vi "MultithreadedUDPReadWriteAnalyze.vi"() -> ()   [LabVIEW 2012]
panel:
  out "regmap":string
  out "power monitoring \ndata string":string
  out "UDP Send Error Initialize":errorcluster
  out "Fresh Register map":bool
  out "Last Command Sent":string
  out "UDP Send Error":errorcluster
  out "Original Register Map":string
  out "Register Map":string
  in  "stop":bool
  out "NumBins":u32
  out "Cnts/Bin":u32
  out "Prof/Hist":u32
  out "Sync":u32
  out "Channel":u32
  out "rTime":u32
  out "frameCntr":u32
  out "UDP Close Error":errorcluster
  out "Profile Byte by Byte":u8[](graph)
  out "Profile":u32[](graph)
  in  "Profile Number":u32=1
  out "Queue close error":errorcluster
  out "Queue Add Data Error":errorcluster
  out "Queue creation error":errorcluster
  out "UDP Read Error":errorcluster
  in  "port":u16=300
  out "UDP Open Error":errorcluster
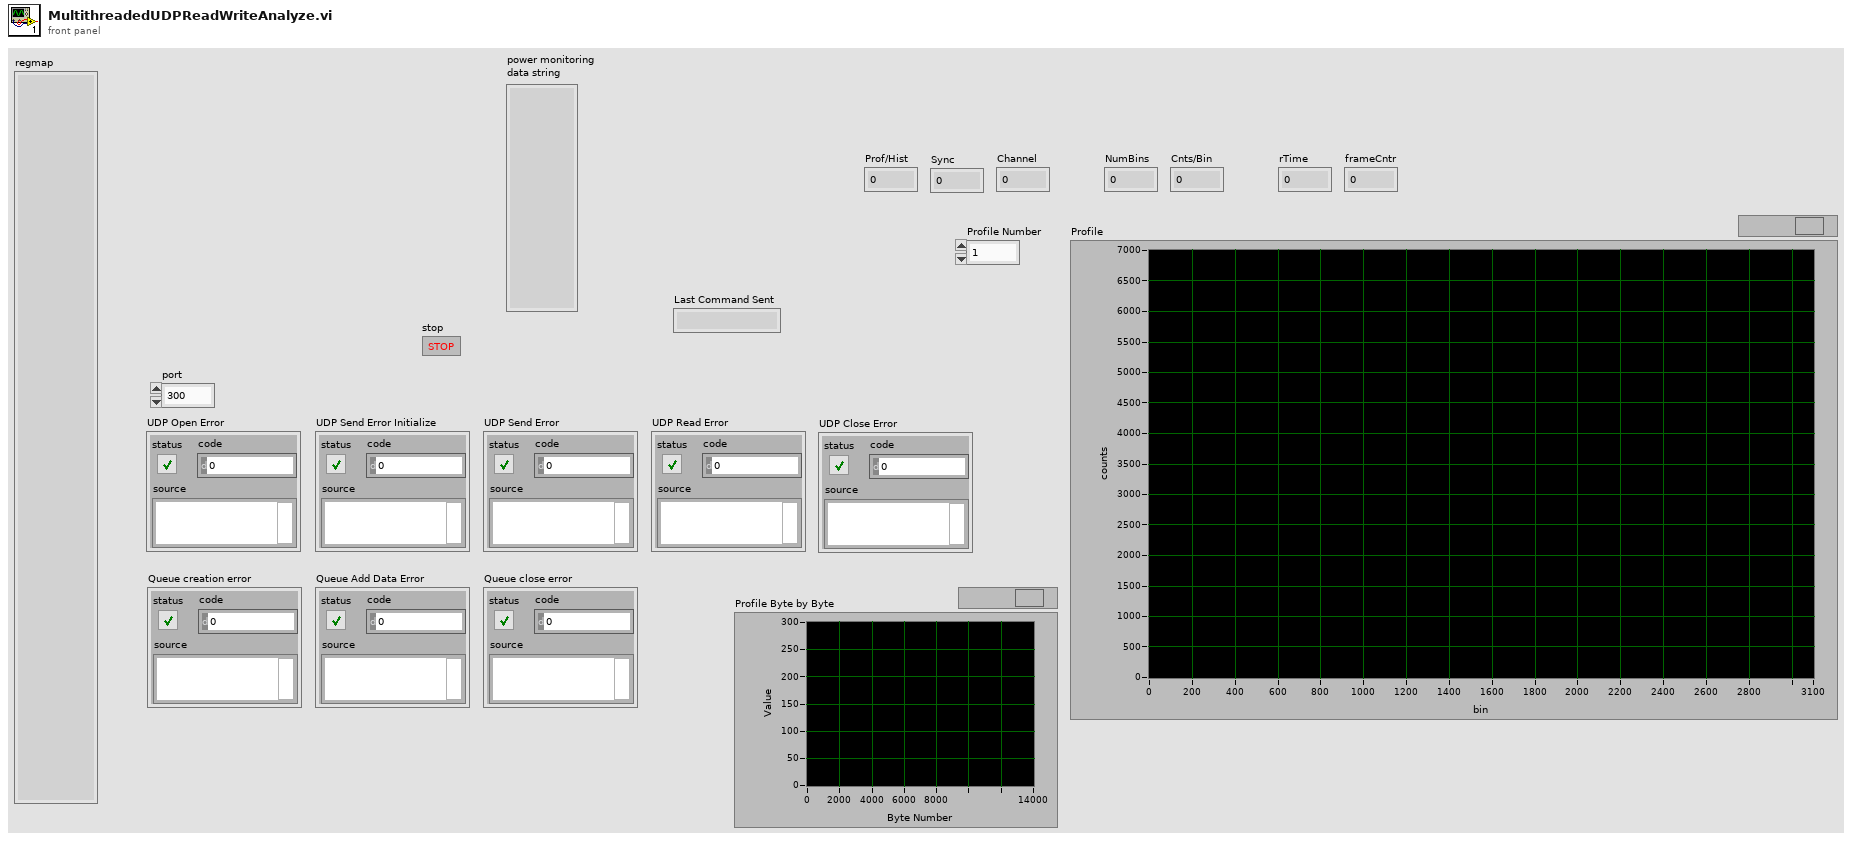
[diagram p1: front panel]
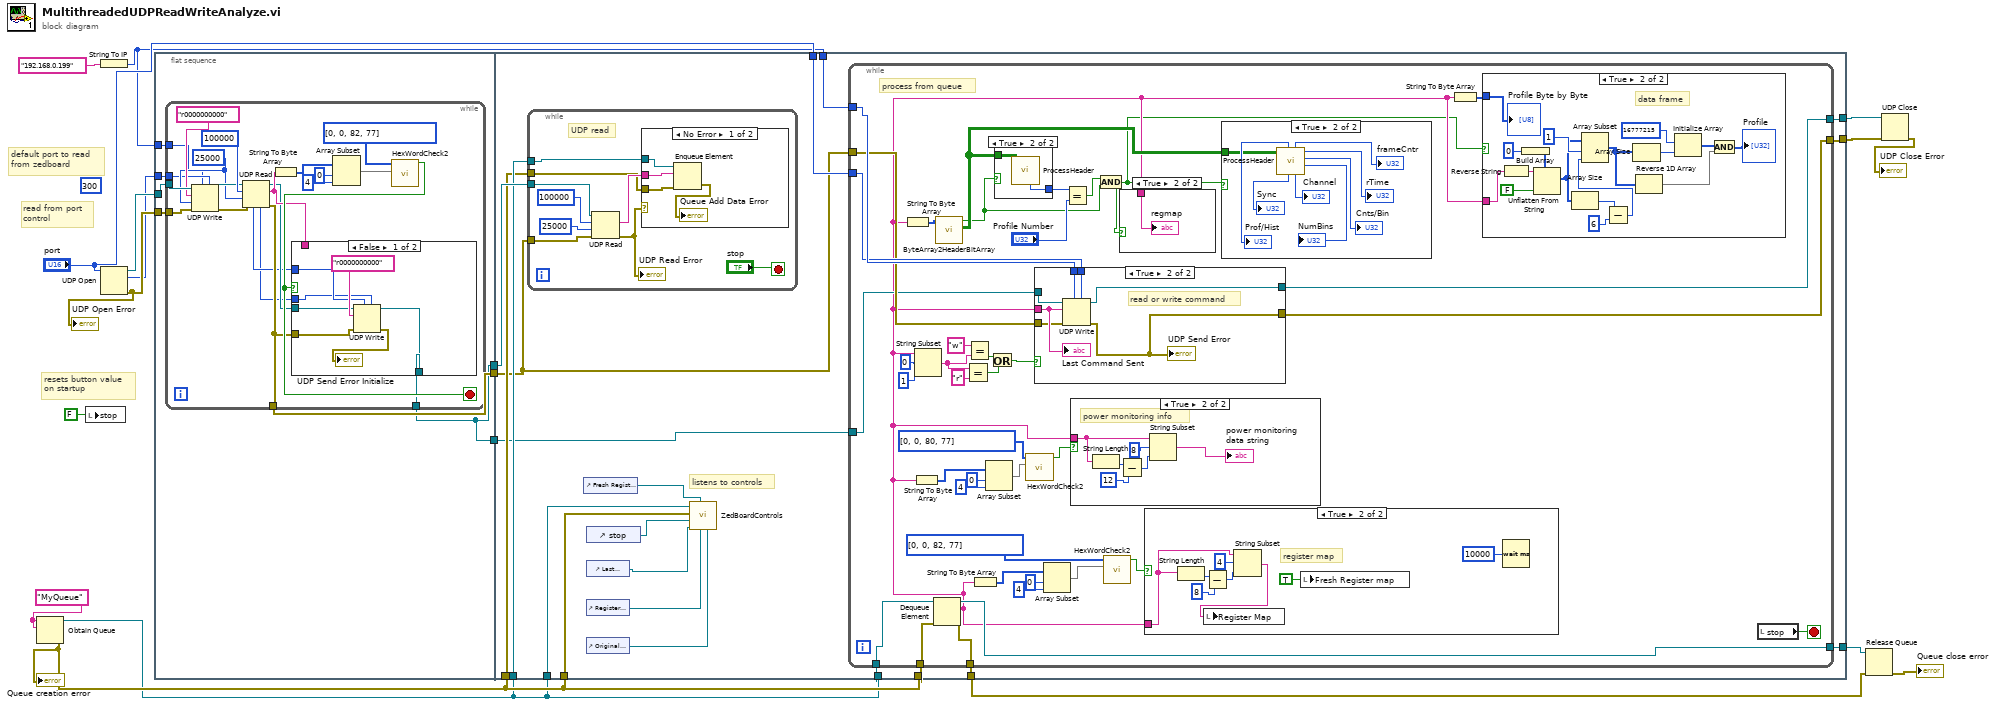
[diagram p0: block diagram]
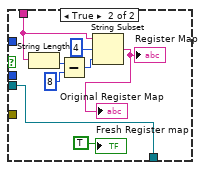
[diagram p2: hidden frame]
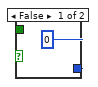
[diagram p7: hidden frame]
diagram:
  w18 = "MyQueue" ("name (unnamed)")
  (unwired) u16 300 ("port")
  # "resets button value \non startup"
  # "default port to read \nfrom zedboard"
  # "read from port\ncontrol"
  n1 = Obtain Queue(name (unnamed)=w18, element data type=w18) -> (queue out=w7:refnum<queue>, error out=w8:errorcluster)  [unwired: 3 in, 1 out]
  "Queue creation error" <- w8
  n2 = local write "stop"(FALSE ("stop")) -> ()
  n3 = String To IP(1:"192.168.0.199" ("name")) -> (0:w1:u32)
  n4 = UDP Open(11:"port") -> (port=w5:refnum<k16>, 0:w6:errorcluster, 2:w2:u16)  [unwired: 4 in]
  "UDP Open Error" <- w6
  n5 = flat-sequence {
    tunnel: [w22] -> w14
    tunnel: [w25] -> w13
    tunnel: w6 -> [w24]
    tunnel: w5 -> [w23]
    tunnel: [w22] -> w3
    tunnel: w2 -> [w21]
    tunnel: w1 -> [w20]
    tunnel: w14 -> [w76]
    tunnel: w7 -> [w75]
    tunnel: w8 -> [w74]
    tunnel: w13 -> [w64]
    tunnel: w7 -> [w73]
    tunnel: [w72] -> w12
    tunnel: [w71] -> w11
    tunnel: w8 -> [w70]
    tunnel: [w69] -> w10
    tunnel: [w68] -> w9
    tunnel: w1 -> [w67]
    tunnel: "port" -> [w66]
    tunnel: w8 -> [w65]
    tunnel: w7 -> [w63]
    tunnel: w3 -> [w62]
    frame #0 {
      n6 = while {
        tunnel: w24 -> [w32]
        tunnel: w23 -> [w33]
        tunnel: [w38] -> w25
        tunnel: [w36] -> w22
        tunnel: w21 -> [w27]
        tunnel: w20 -> [w26]
        stop <- w44 stop-if-true
        w28 = 25000 ("timeout ms (25000)")
        n7 = UDP Write(address=w26, port or service name=w27, connection ID=w33, data in="r0000000000", 8:w32, 9:w28) -> (error out=w31:errorcluster, 3:w30:refnum<k16>)
        n8 = UDP Read(connection ID=w30, max size (548)=100000, timeout ms (25000)=w28, 8:w31) -> (data out=w39:string, error out=w38:errorcluster, 3:w37:refnum<k16>, 4:w34:u16, 6:w35:u32)
        n9 = String To Byte Array(string=w39) -> (unsigned byte array=w43:u8[])
        n10 = Array Subset(array=w43, index=0, length=4) -> (w42:u8[])
        n11 = call "HexWordCheck2.vi"("array"=w42, "Input Array"=u8[] [0, 0, 82, 77]) -> ("Boolean"=w44:bool)  [unwired: 9 in]
        n12 = case shown="False" w44 {
          tunnel: w39 -> [_ w57]
          tunnel: w34 -> [w47 _]
          tunnel: w35 -> [w48 _]
          tunnel: w38 -> [w51 _]
          tunnel: w37 -> [w50 w54]
          tunnel: [w49 w54] -> w36
          frame False {
            n13 = UDP Write(address=w48, port or service name=w47, connection ID=w50, data in="r0000000000", 8:w51) -> (error out=→"UDP Send Error Initialize":errorcluster, 3:w49:refnum<k16>)  [unwired: 1 in]
          }
          frame True {
            n14 = String Length(string=w57) -> (length=w59:i32)
            n15 = Subtract(x=w59, y=8) -> (x-y=w61:i32)
            n16 = String Subset(string=w57, offset (0)=4, length (rest)=w61) -> (substring=→"Register Map" →"Original Register Map":string)
            "Fresh Register map" <- TRUE ("Fresh Register map")
          }
        }
      }
    }
    frame #1 {
      # "listens to controls"
      n17 = while {
        tunnel: w75 -> [w177]
        tunnel: w74 -> [w178]
        tunnel: w64 -> [w180]
        tunnel: w76 -> [w174]
        stop <- "stop" stop-if-true
        # "UDP read"
        n18 = UDP Read(connection ID=w174, max size (548)=100000, timeout ms (25000)=25000, 8:w180) -> (data out=w179:string, error out=w176:errorcluster)  [unwired: 3 out]
        "UDP Read Error" <- w176
        n19 = case shown="No Error" w176 {
          tunnel: w179 -> [w186 _]
          tunnel: w178 -> [w185 _]
          tunnel: w177 -> [w184 _]
          frame No Error {
            n20 = Enqueue Element(queue=w184, element=w186, error in (no error)=w185) -> (error out=→"Queue Add Data Error":errorcluster)  [unwired: 1 in, 2 out]
          }
          frame Error {
          }
        }
      }
      n21 = control-ref of="Fresh Register map"() -> (w81:refnum<vi>)
      n22 = control-ref of="stop"() -> (w79:refnum<vi>)
      n23 = control-ref of="Last Command Sent"() -> (w80:refnum<vi>)
      n24 = control-ref of="Register Map"() -> (w77:refnum<vi>)
      n25 = control-ref of="Original Register Map"() -> (w78:refnum<vi>)
      n26 = call "ZedBoardControls.vi"("Register Map\nDefaults"=w78, "Register Map\nRead Ref"=w77, "NewRegMapReady"=w81, "Last Command\nSent Ref"=w80, "Stop Loop \nRef"=w79, "error out"=w65, "queue out"=w73) -> ()  [unwired: 5 in]
      n27 = while {
        tunnel: w70 -> [w121]
        tunnel: [w119] -> w68
        tunnel: [w120] -> w69
        tunnel: [w115] -> w72
        tunnel: [w114] -> w71
        tunnel: w64 -> [w116]
        tunnel: w67 -> [w118]
        tunnel: w66 -> [w117]
        tunnel: w63 -> [w112]
        tunnel: w62 -> [w111]
        stop <- w113 stop-if-true
        # "process from queue"
        n28 = Dequeue Element(queue=w112, error in (no error)=w121) -> (queue out=w119:refnum<queue>, element=w86:string, error out=w120:errorcluster)  [unwired: 1 in, 1 out]
        n29 = String To Byte Array(string=w86) -> (unsigned byte array=w97:u8[])
        n30 = String To Byte Array(string=w86) -> (unsigned byte array=w90:u8[])
        n31 = String Subset(string=w86, offset (0)=0, length (rest)=1 ("length (rest)")) -> (substring=w107:string)
        n32 = call "ByteArray2HeaderBitArray.vi"("Input Byte Array"=w97) -> ("Header Array"=w87:bool[][], "Found Header"=w85:bool)  [unwired: 9 in]
        n33 = Equal?(x=w107, y="r") -> (x = y?=w103:bool)
        n34 = Equal?(x="w", y=w107) -> (x = y?=w102:bool)
        n35 = String To Byte Array(string=w86) -> (unsigned byte array=w82:u8[])
        n36 = Array Subset(array=w90, index=0, length=4) -> (w89:u8[])
        n37 = Or(x=w102, y=w103) -> (x .or. y?=w101:bool)
        n38 = case shown="True" w85 {
          tunnel: w87 -> [_ w156]
          tunnel: [u32 0 ("Channel") w155] -> w99
          frame False {
          }
          frame True {
            n39 = call "ProcessHeader.vi"("Array"=w156) -> ("Channel"=w155:u32)  [unwired: 4 in, 6 out]
          }
        }
        n40 = call "HexWordCheck2.vi"("array"=w89, "Input Array"=u8[] [0, 0, 80, 77] ("array")) -> ("Boolean"=w88:bool)  [unwired: 9 in]
        n41 = case shown="True" w101 {
          tunnel: w86 -> [_ w165]
          tunnel: w118 -> [_ w164]
          tunnel: w117 -> [_ w163]
          tunnel: w111 -> [w158 w162]
          tunnel: w116 -> [w157 w161]
          tunnel: [w158 w160] -> w115
          tunnel: [w157 w159] -> w114
          frame False {
          }
          frame True {
            # "read or write command"
            n42 = UDP Write(address=w164, port or service name=w163, connection ID=w162, data in=w165, 8:w161) -> (error out=w159:errorcluster, 3:w160:refnum<k16>)  [unwired: 1 in]
            "UDP Send Error" <- w159
            "Last Command Sent" <- w165
          }
        }
        n43 = Array Subset(array=w82, index=0, length=4) -> (w83:u8[])
        n44 = Equal?(x=w99, y="Profile Number") -> (x = y?=w98:bool)
        n45 = case shown="True" w88 {
          tunnel: w86 -> [_ w124]
          frame False {
          }
          frame True {
            # "power monitoring info"
            n46 = String Length(string=w124) -> (length=w125:i32)
            n47 = Subtract(x=w125, y=12) -> (x-y=w127:i32)
            n48 = String Subset(string=w124, offset (0)=8, length (rest)=w127) -> (substring=→"power monitoring \ndata string":string)
          }
        }
        n49 = And(x=w98, y=w85) -> (x .and. y?=w84:bool)
        n50 = call "HexWordCheck2.vi"("array"=w83, "Input Array"=u8[] [0, 0, 82, 77] ("array")) -> ("Boolean"=w109:bool)  [unwired: 9 in]
        n51 = case shown="True" w84 {
          tunnel: w86 -> [_ w122]
          frame False {
          }
          frame True {
            "regmap" <- w122
          }
        }
        n52 = case shown="True" w109 {
          tunnel: w86 -> [_ w170]
          frame False {
          }
          frame True {
            # "register map"
            n53 = String Length(string=w170) -> (length=w173:i32)
            n54 = Subtract(x=w173, y=8) -> (x-y=w172:i32)
            n55 = String Subset(string=w170, offset (0)=4, length (rest)=w172) -> (substring=w171:string)
            n56 = local write "Register Map"(w171) -> ()
            n57 = local write "Fresh Register map"(TRUE ("Fresh Register map")) -> ()
            n58 = Wait (ms)(milliseconds to wait=u32 10000) -> ()  [unwired: 1 out]
          }
        }
        n59 = case shown="True" w84 {
          tunnel: w87 -> [_ w147]
          frame False {
          }
          frame True {
            n60 = call "ProcessHeader.vi"("Array"=w147) -> ("Number of Bins"=→"NumBins":u32, "Counts Per Bin"=→"Cnts/Bin":u32, "rTime"=→"rTime":u32, "Channel"=→"Channel":u32, "Frame Counter"=→"frameCntr":u32, "Sync"=→"Sync":u32, "Profiles Per Hist"=→"Prof/Hist":u32)  [unwired: 4 in]
          }
        }
        n61 = String To Byte Array(string=w86) -> (unsigned byte array=w96:u8[])
        n62 = case shown="True" w84 {
          tunnel: w96 -> [_ w131]
          tunnel: w86 -> [_ w130]
          frame False {
          }
          frame True {
            # "data frame"
            n63 = Reverse String(1:w130) -> (0:w139:string)
            n64 = Build Array(u32 0) -> (w133:u32[])
            n65 = Unflatten From String(type=w133, binary string=w139, data includes array or string size? (T)=FALSE) -> (value=w135:u32[])  [unwired: 2 in, 2 out]
            n66 = Array Size(array=w135) -> (size(s)=w136:i32)
            n67 = Subtract(x=w136, y=6) -> (x-y=w129:i32)
            n68 = Array Subset(array=w135, index=1, length=w129) -> (w140:u32[])
            n69 = Array Size(array=w140) -> (size(s)=w143:i32)
            n70 = Reverse 1D Array(array=w140) -> (reversed array=w141:u32[])
            n71 = Initialize Array(u32 16777215 ("x*2^n"), w143) -> (w142:u32[])
            n72 = And(x=w142, y=w141) -> (x .and. y?=→"Profile":u32[])
            "Profile Byte by Byte" <- w131
          }
        }
        n73 = local read "stop"() -> (w113:bool)
      }
    }
  }
  n74 = Release Queue(queue=w9, error in (no error)=w10) -> (error out=→"Queue close error":errorcluster)  [unwired: 1 in, 2 out]
  n75 = UDP Close(connection ID=w12, 8:w11) -> (error out=→"UDP Close Error":errorcluster)  [unwired: 1 out]
